vi "take_data (SubVI).vi"(2 "Synth_sync":bool, 3 "channel settings":T2={"samples per channel"=1000.0, "sampling rate"=1000.0, "data task"="", "Clock src"=""} {"sampling rate" format="%0.2f"}) -> (0 "data tasks":T1, 1 "Actual Sample Rate":dbl=10000.0 format="%0.2f")   [LabVIEW 2018]
uses:
  <vilib>/DAQmx/create/channels.llb/DAQmx Create Channel (AI-Voltage-Basic).vi
  <vilib>/DAQmx/configure/timing.llb/DAQmx Timing (Sample Clock).vi
  <vilib>/DAQmx/configure/trigger.llb/DAQmx Start Trigger (Digital Edge).vi
  <resource>/objmgr/daqmx.rc
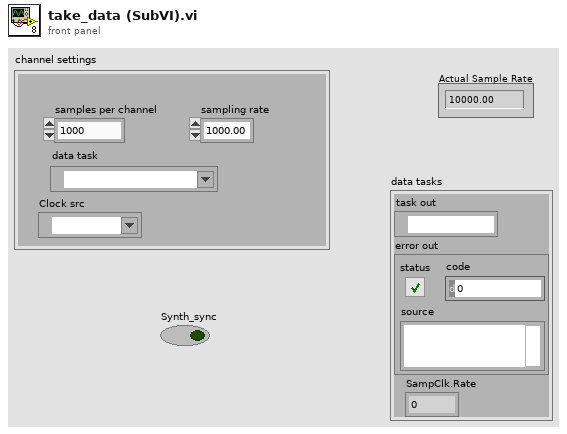
[diagram p1: front panel]
types:
  T1 = cluster{"task out":refnum<k21>, "error out":errorcluster, "SampClk.Rate":dbl}
  T2 = cluster{"samples per channel":dbl, "sampling rate":dbl, "data task":tag, "Clock src":tag}
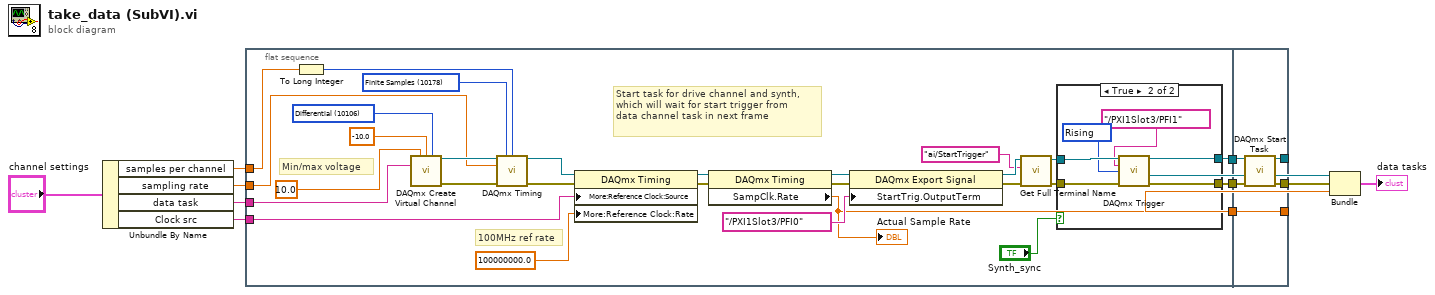
[diagram p0: block diagram]
diagram:
  n1 = Unbundle By Name("channel settings") -> ("samples per channel"=w7:dbl, "sampling rate"=w10:dbl, "data task"=w11:tag, "Clock src"=w6:tag)
  n2 = flat-sequence {
    tunnel: w11 -> [w27]
    tunnel: w10 -> [w22]
    tunnel: w7 -> [w19]
    tunnel: [w16] -> w3
    tunnel: [w14] -> w2
    tunnel: [w21] -> w1
    tunnel: w6 -> [w20]
    tunnel: w3 -> [w53]
    tunnel: w2 -> [w52]
    tunnel: [w51] -> w9
    tunnel: [w50] -> w8
    tunnel: [w49] -> w5
    tunnel: w1 -> [w49]
    frame #0 {
      w28 = 10106 items=["default"=-1, "RSE"=10083, "NRSE"=10078, "Differential"=10106, "Pseudodifferential"=12529] ("input terminal configuration")
      w24 = 10178 items=["Finite Samples"=10178, "Continuous Samples"=10123, "Hardware Timed Single Point"=12522] ("sample mode")
      # "Start task for drive channel and synth,\nwhich will wait for start trigger from \ndata channel task in next frame"
      # "100MHz ref rate"
      # "Min/max voltage"
      n3 = To Long Integer(number=w19) -> (32bit integer=w18:i32)
      n4 = call-poly <vilib>:"DAQmx Create Virtual Channel.vi"("maximum value"=10.0, "minimum value"=-10.0, "input terminal configuration"=w28, "physical channels"=w27) -> ("task out"=w29:refnum<k21>, "error out"=w30:errorcluster)  [unwired: 10 in]
      n5 = call-poly <vilib>:"DAQmx Timing.vi"("task/channels in"=w29, "sample mode"=w24, "samples per channel"=w18, "rate"=w22, "error in"=w30) -> ("task out"=w31:refnum<k21>, "error out"=w32:errorcluster)  [unwired: 9 in]
      n6 = property class="DAQmx Timing"(reference=w31, error in=w32, "More:Reference Clock:Source"=w20, "More:Reference Clock:Rate"=100000000.0 ("RefClk.Rate")) -> (reference out=w33:refnum<k21>, error out=w34:errorcluster)
      n7 = property class="DAQmx Timing"(reference=w33, error in=w34) -> (reference out=w36:refnum<k21>, error out=w38:errorcluster, "SampClk.Rate"=w21:dbl)
      "Actual Sample Rate" <- w21
      n8 = property class="DAQmx Export Signal"(reference=w36, error in=w38, "StartTrig.OutputTerm"=tag "/PXI1Slot3/PFI0") -> (reference out=w37:refnum<k21>, error out=w39:errorcluster)
      n9 = call "Get Full Terminal Name.vi"("error in (no error)"=w39, "Local Terminal Name"="ai/StartTrigger", "task/channels in"=w37) -> ("error out"=w15:errorcluster, "task out"=w17:refnum<k21>)  [unwired: 6 in, 1 out]
      n10 = case shown="True" "Synth_sync" {
        tunnel: w17 -> [w41 w48]
        tunnel: [w41 w47] -> w16
        tunnel: w15 -> [w42 w44]
        tunnel: [w42 w43] -> w14
        frame False {
        }
        frame True {
          w45 = 10280 items=["Rising"=10280, "Falling"=10171] ("edge")
          n11 = call-poly <vilib>:"DAQmx Trigger.vi"("task/channels in"=w48, "source"=tag "/PXI1Slot3/PFI1", "edge"=w45, "error in"=w44) -> ("task out"=w47:refnum<k21>, "error out"=w43:errorcluster)  [unwired: 10 in]
        }
      }
    }
    frame #1 {
      n12 = call <vilib>:"DAQmx Start Task.vi"("task/channels in"=w53, "error in"=w52) -> ("task out"=w51:refnum<k21>, "error out"=w50:errorcluster)  [unwired: 12 in]
    }
  }
  n13 = Bundle("task out"=w9, "error out"=w8, "SampClk.Rate"=w5) -> (→"data tasks":T1)  [unwired: 1 in]
